vi "setpoint.vi"(9 "fine_approach\nsetpoint":dbl=0.9, 10 "quick_approach\nsetpoint":dbl=0.99, 11 "Coarse Approach.lvclass":refnum<class "Coarse Approach.lvclass">) -> (1 "free amplitude":dbl, 2 "output cluster":T1, 3 "Coarse Approach.lvclass":refnum<class "Coarse Approach.lvclass">)   [LabVIEW 2020, in "Coarse Approach.lvclass"]
uses:
  Coarse Approach.lvclass
  Coarse Approach.lvclass/Coarse Approach.ctl
panel:
  in  "input cluster":T1
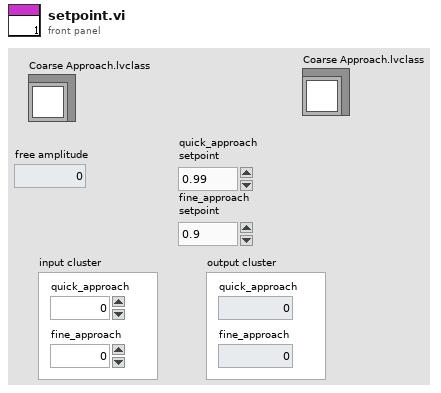
[diagram p1: front panel]
types:
  T1 = cluster{"quick_approach":dbl, "fine_approach":dbl}
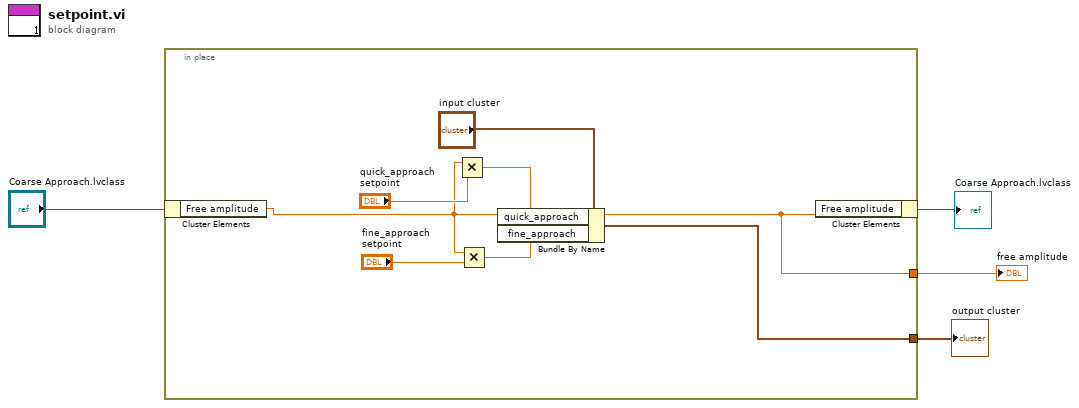
[diagram p0: block diagram]
diagram:
  n1 = in-place {
    in-place-border: [w6] -> w3
    in-place-border: [w5] -> w1
    n2 = in-place-cluster #1("Coarse Approach.lvclass") -> ("Free amplitude"=w5:dbl)
    n3 = Multiply(x=w5, y="quick_approach\nsetpoint") -> (x*y=w9:dbl)
    n4 = Multiply(x=w5, y="fine_approach\nsetpoint") -> (x*y=w8:dbl)
    n5 = Bundle By Name(cluster="input cluster", "quick_approach"=w9, "fine_approach"=w8) -> (w6:T1)
    n6 = in-place-cluster #1("Free amplitude"=w5) -> (→"Coarse Approach.lvclass":refnum<class "Coarse Approach.lvclass">)
  }
  "output cluster" <- w3
  "free amplitude" <- w1
